vi "write_to_csv.vi"() -> ()   [LabVIEW 2024]
uses:
  <vilib>/Utility/file.llb/Write Delimited Spreadsheet (string).vi
panel:
  in  "Person Details":T1
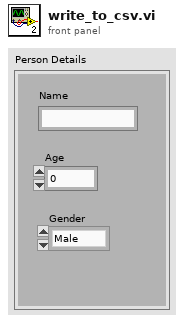
[diagram p1: front panel]
types:
  T1 = cluster{"Name":string, "Age":dbl, "Gender":enum16{"Male", "Female"}}
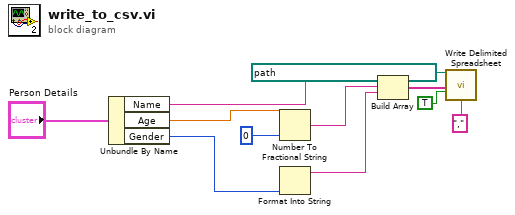
[diagram p0: block diagram]
diagram:
  n1 = Unbundle By Name("Person Details") -> ("Name"=w7:string, "Age"=w10:dbl, "Gender"=w8:enum16{"Male", "Female"})
  n2 = Number To Fractional String(number=w10, precision (6)=0) -> (F-format string=w6:string)  [unwired: 2 in]
  n3 = Format Into String(w8) -> (resulting string=w5:string)  [unwired: 3 in, 1 out]
  n4 = Build Array(w7, w6, w5) -> (w4:string[])
  n5 = call-poly <vilib>:"Write Delimited Spreadsheet.vi"("file path (dialog if empty)"=path "C:/Users/Eylül Öztek/Desktop/staj notlar/2 - 02.07.2024/detail.csv", "1D data"=w4, "append to file? (new file:F)"=TRUE, "delimiter (\\t)"="," ("delimiter (\\t)")) -> ()  [unwired: 10 in, 2 out]
